vi "Bass Subvi2.vi"(0 "Image Dst Out":T2, 1 "Blue Bass 2":T1={"Global Rectangle"=[192, 292, 199, 386], "Contours"=[{"ID"=enum."External", "Type"=2, "Coordinates"=[192, 385, 198, 292]}]} {"Contours"."Type" items=["No Selection", "Point", "Line", "Rectangle", "Oval", "Polygon", "Freehand Region", "Annulus", "Unused2", "Unused3", "Broken Line", "Freehand Line", "Rotated Rectangle"]}, 2 "Yellow Bass 2":T1={"Global Rectangle"=[160, 295, 175, 378], "Contours"=[{"ID"=enum."External", "Type"=2, "Coordinates"=[160, 377, 174, 295]}]} {"Contours"."Type" items=["No Selection", "Point", "Line", "Rectangle", "Oval", "Polygon", "Freehand Region", "Annulus", "Unused2", "Unused3", "Broken Line", "Freehand Line", "Rotated Rectangle"]}, 3 "Green Bass 2":T1={"Global Rectangle"=[100, 292, 131, 371], "Contours"=[{"ID"=enum."External", "Type"=2, "Coordinates"=[100, 370, 130, 292]}]} {"Contours"."Type" items=["No Selection", "Point", "Line", "Rectangle", "Oval", "Polygon", "Freehand Region", "Annulus", "Unused2", "Unused3", "Broken Line", "Freehand Line", "Rotated Rectangle"]}, 4 "Red Bass 2":T1={"Global Rectangle"=[129, 294, 154, 376], "Contours"=[{"ID"=enum."External", "Type"=2, "Coordinates"=[129, 375, 153, 294]}]} {"Contours"."Type" items=["No Selection", "Point", "Line", "Rectangle", "Oval", "Polygon", "Freehand Region", "Annulus", "Unused2", "Unused3", "Broken Line", "Freehand Line", "Rotated Rectangle"]}, 5 "Orange Bass 2":T1={"Global Rectangle"=[220, 302, 227, 392], "Contours"=[{"ID"=enum."External", "Type"=2, "Coordinates"=[226, 391, 220, 302]}]} {"Contours"."Type" items=["No Selection", "Point", "Line", "Rectangle", "Oval", "Polygon", "Freehand Region", "Annulus", "Unused2", "Unused3", "Broken Line", "Freehand Line", "Rotated Rectangle"]}, 8 "error out":errorcluster) -> (9 "Orange Bass LED":bool, 11 "Red Bass LED":bool, 13 "Green Bass LED":bool, 15 "Yellow Bass LED":bool, 19 "Blue Bass LED":bool, 27 "error out 2":errorcluster)   [LabVIEW 2009]
uses:
  <vilib>/vision/Image Controls.llb/IMAQ Image.ctl
  <vilib>/Analysis/3filter.llb/Filter Passband Type.ctl
  <vilib>/Analysis/3filter.llb/Butterworth Filter (DBL).vi
  <vilib>/Analysis/NI_AALBase.lvlib
  <vilib>/vision/NI_Vision_Development_Module.lvlib
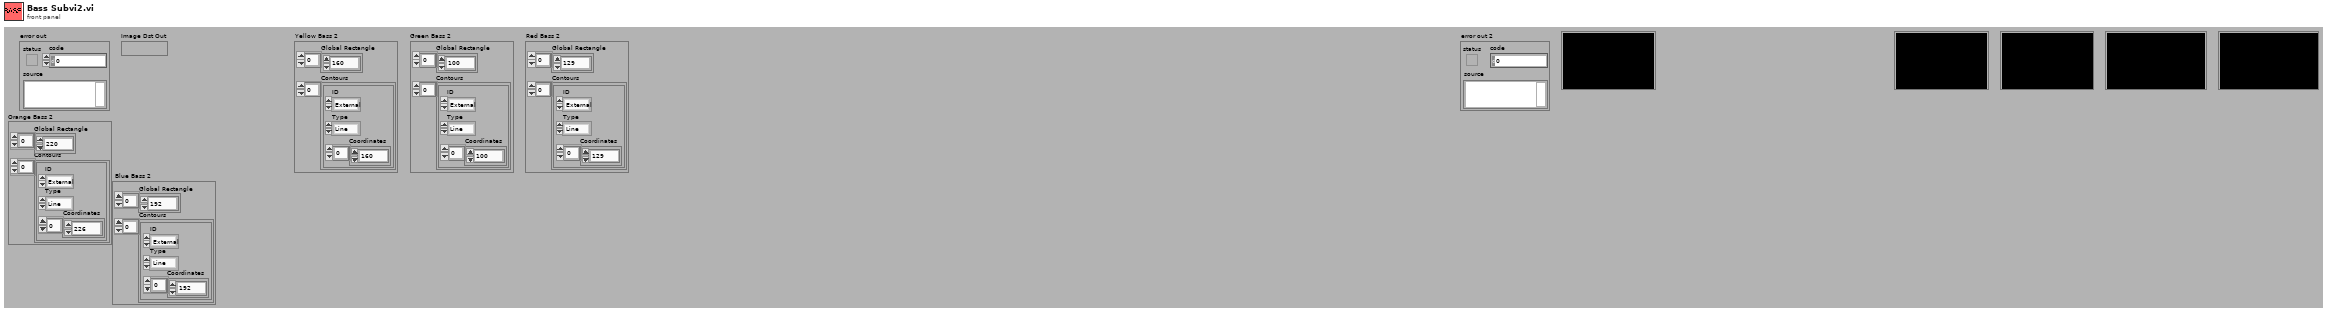
[diagram p1: front panel]
types:
  T1 = cluster{"Global Rectangle":i32[], "Contours":cluster{"ID":enum32{"External", "Internal"}, "Type":u32, "Coordinates":i32[]}[]}
  T2 = typedef "IMAQ Image.ctl" = refnum<image>
  T3 = typedef "NI_AALBase.lvlib/Filter Passband Type.ctl" = enum32{"Lowpass", "Highpass", "Bandpass", "Bandstop"}
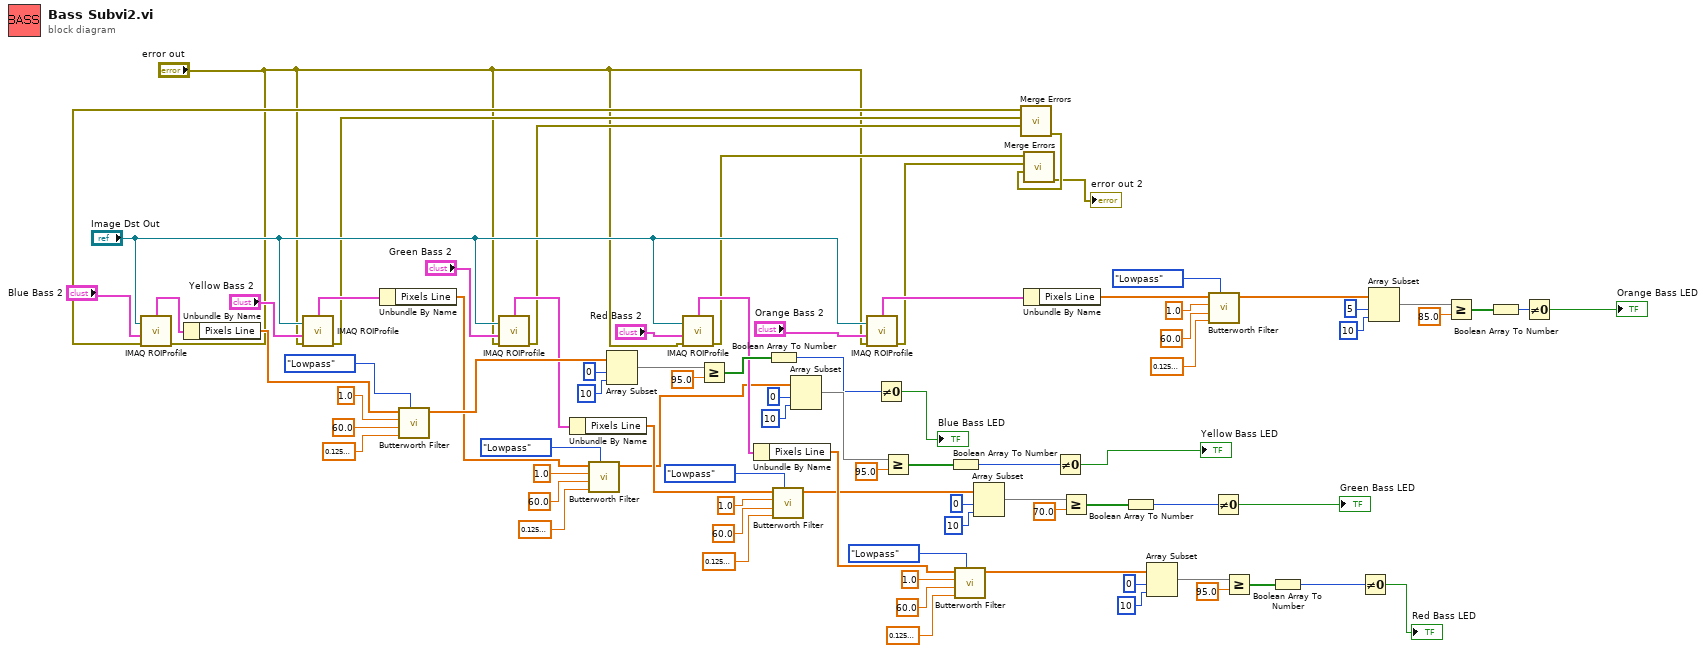
[diagram p0: block diagram]
diagram:
  n1 = call "IMAQ ROIProfile"("error in (no error)"="error out", "ROI Descriptor"="Blue Bass 2", "Image"="Image Dst Out") -> ("error out"=w8:errorcluster, "ROI Graph"=w34:cluster{"x0":sgl, "dx":sgl, "Pixels Line":sgl[]})  [unwired: 4 out]
  n2 = Unbundle By Name(w34) -> ("Pixels Line"=w12:sgl[])
  n3 = call "IMAQ ROIProfile"("error in (no error)"="error out", "ROI Descriptor"="Yellow Bass 2", "Image"="Image Dst Out") -> ("error out"=w7:errorcluster, "ROI Graph"=w31:cluster{"x0":sgl, "dx":sgl, "Pixels Line":sgl[]})  [unwired: 4 out]
  n4 = Unbundle By Name(w31) -> ("Pixels Line"=w28:sgl[])
  n5 = call-poly <vilib>:"Butterworth Filter.vi"("filter type"=Filter_Passband_Type."Lowpass", "low cutoff freq: fl"=0.12500000000000006 ("low 2"), "high cutoff freq: fh"=60.0 ("high 8"), "sampling freq: fs"=1.0 ("sampling  8"), "X"=w12) -> ("Filtered X"=w48:dbl[])  [unwired: 3 in, 1 out]
  n6 = call "IMAQ ROIProfile"("error in (no error)"="error out", "ROI Descriptor"="Green Bass 2", "Image"="Image Dst Out") -> ("error out"=w6:errorcluster, "ROI Graph"=w36:cluster{"x0":sgl, "dx":sgl, "Pixels Line":sgl[]})  [unwired: 4 out]
  n7 = Unbundle By Name(w36) -> ("Pixels Line"=w39:sgl[])
  n8 = call-poly <vilib>:"Butterworth Filter.vi"("filter type"=Filter_Passband_Type."Lowpass", "low cutoff freq: fl"=0.12500000000000006 ("low  7"), "high cutoff freq: fh"=60.0 ("high 7"), "sampling freq: fs"=1.0 ("sampling 7"), "X"=w28) -> ("Filtered X"=w32:dbl[])  [unwired: 3 in, 1 out]
  n9 = Array Subset(array=w48, index=0, length=10) -> (w18:dbl[])
  n10 = call "IMAQ ROIProfile"("error in (no error)"="error out", "ROI Descriptor"="Red Bass 2", "Image"="Image Dst Out") -> ("error out"=w5:errorcluster, "ROI Graph"=w60:cluster{"x0":sgl, "dx":sgl, "Pixels Line":sgl[]})  [unwired: 4 out]
  n11 = Greater Or Equal?(x=w18, y=95.0) -> (x >= y?=w83:bool[])
  n12 = Unbundle By Name(w60) -> ("Pixels Line"=w57:sgl[])
  n13 = Boolean Array To Number(Boolean array=w83) -> (number=w20:u32)
  n14 = call-poly <vilib>:"Butterworth Filter.vi"("filter type"=Filter_Passband_Type."Lowpass", "low cutoff freq: fl"=0.12500000000000006 ("low  6"), "high cutoff freq: fh"=60.0 ("high 6"), "sampling freq: fs"=1.0 ("sampling 6"), "X"=w39) -> ("Filtered X"=w35:dbl[])  [unwired: 3 in, 1 out]
  n15 = Array Subset(array=w32, index=0, length=10) -> (w23:dbl[])
  n16 = call "IMAQ ROIProfile"("error in (no error)"="error out", "ROI Descriptor"="Orange Bass 2", "Image"="Image Dst Out") -> ("error out"=w4:errorcluster, "ROI Graph"=w66:cluster{"x0":sgl, "dx":sgl, "Pixels Line":sgl[]})  [unwired: 4 out]
  n17 = Not Equal To 0?(x=w20) -> (x != 0?=→"Blue Bass LED":bool)
  n18 = Greater Or Equal?(x=w23, y=95.0) -> (x >= y?=w25:bool[])
  n19 = Boolean Array To Number(Boolean array=w25) -> (number=w26:u32)
  n20 = call-poly <vilib>:"Butterworth Filter.vi"("filter type"=Filter_Passband_Type."Lowpass", "low cutoff freq: fl"=0.12500000000000006 ("low  5"), "high cutoff freq: fh"=60.0 ("high 5"), "sampling freq: fs"=1.0 ("sampling 5"), "X"=w57) -> ("Filtered X"=w61:dbl[])  [unwired: 3 in, 1 out]
  n21 = Array Subset(array=w35, index=0, length=10) -> (w44:dbl[])
  n22 = call <vilib>:"Merge Errors.vi"("error in 3 (no error)"=w6, "error in 2 (no error)"=w7, "error in 1 (no error)"=w8) -> ("error out"=w3:errorcluster)  [unwired: 4 in]
  n23 = call <vilib>:"Merge Errors.vi"("error in 3 (no error)"=w3, "error in 2 (no error)"=w4, "error in 1 (no error)"=w5) -> ("error out"=→"error out 2":errorcluster)  [unwired: 4 in]
  n24 = Unbundle By Name(w66) -> ("Pixels Line"=w69:sgl[])
  n25 = Not Equal To 0?(x=w26) -> (x != 0?=→"Yellow Bass LED":bool)
  n26 = Greater Or Equal?(x=w44, y=70.0) -> (x >= y?=w42:bool[])
  n27 = Boolean Array To Number(Boolean array=w42) -> (number=w41:u32)
  n28 = Array Subset(array=w61, index=0, length=10) -> (w52:dbl[])
  n29 = call-poly <vilib>:"Butterworth Filter.vi"("filter type"=Filter_Passband_Type."Lowpass", "low cutoff freq: fl"=0.12500000000000006 ("low  8"), "high cutoff freq: fh"=60.0 ("high 9"), "sampling freq: fs"=1.0 ("sampling 8"), "X"=w69) -> ("Filtered X"=w65:dbl[])  [unwired: 3 in, 1 out]
  n30 = Not Equal To 0?(x=w41) -> (x != 0?=→"Green Bass LED":bool)
  n31 = Greater Or Equal?(x=w52, y=95.0) -> (x >= y?=w54:bool[])
  n32 = Boolean Array To Number(Boolean array=w54) -> (number=w55:u32)
  n33 = Not Equal To 0?(x=w55) -> (x != 0?=→"Red Bass LED":bool)
  n34 = Array Subset(array=w65, index=5, length=10) -> (w74:dbl[])
  n35 = Greater Or Equal?(x=w74, y=85.0) -> (x >= y?=w72:bool[])
  n36 = Boolean Array To Number(Boolean array=w72) -> (number=w71:u32)
  n37 = Not Equal To 0?(x=w71) -> (x != 0?=→"Orange Bass LED":bool)
